vi "Get Step Information From Sequencer Configuration.vi"(10 "LstBox Refnum":refnum<vi>, 11 "Sequencer Module configuration in":refnum<class "Sequencer Module configuration.lvclass">) -> (0 "error out":errorcluster, 3 "Array":string[][](array[string]))   [LabVIEW 2015]
uses:
  module/configuration/Sequencer Module configuration.lvclass
  module/configuration/Sequencer Module configuration.lvclass/Sequencer Module configuration.ctl
  module/configuration/Read Lines.vi
  classes/Sequence/Config/Sequence Config.lvclass
  classes/Step/Config/Step Config.lvclass
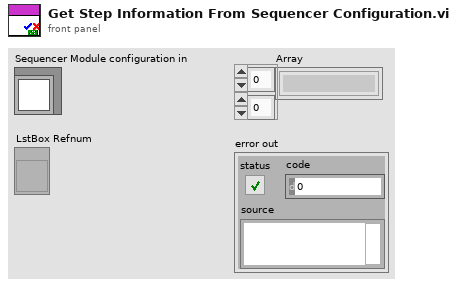
[diagram p1: front panel]
types:
  T1 = typedef "Sequencer Module configuration.lvclass/Line.ctl" = cluster{"Sequence":refnum<class "Sequence Config.lvclass">}
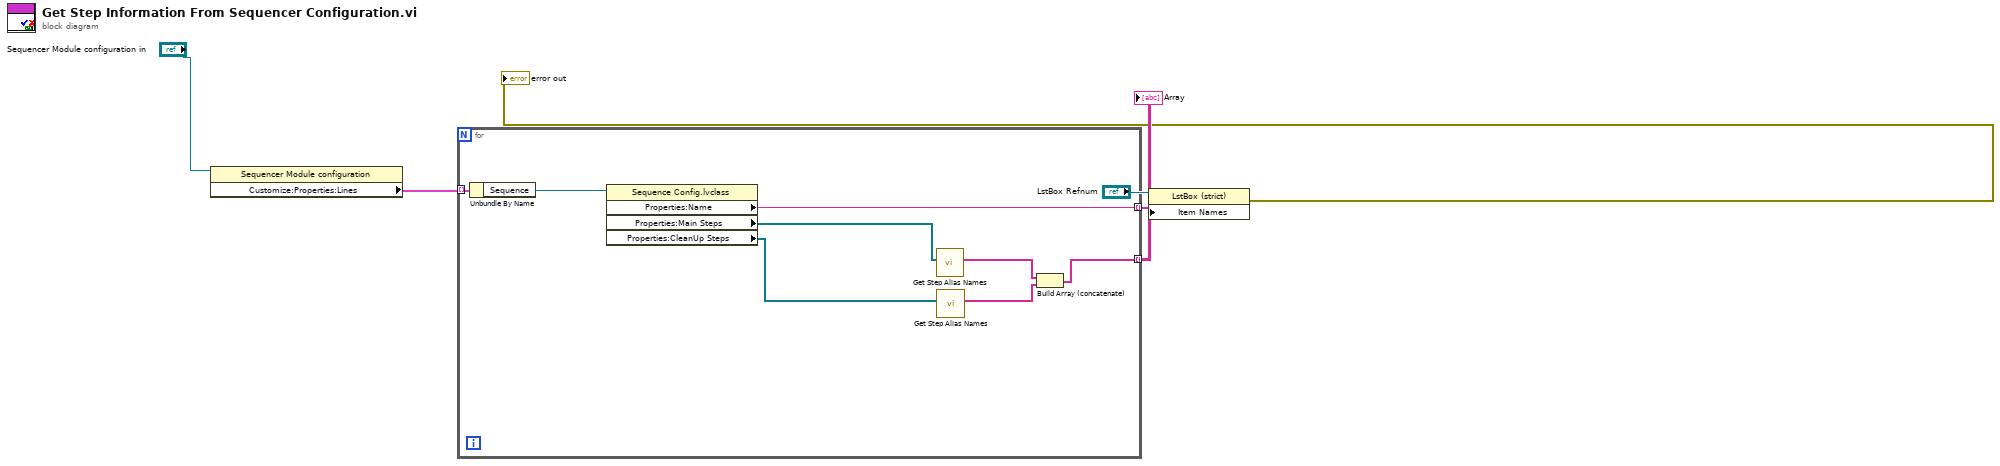
[diagram p0: block diagram]
diagram:
  n1 = property class="Sequencer Module configuration"(reference="Sequencer Module configuration in") -> ("Customize:Properties:Lines"=w3:T1[])  [unwired: 1 in, 2 out]
  n2 = for {
    tunnel: w3 -> [w14] mode=indexing
    tunnel: [w10] -> w4 mode=indexing
    tunnel: [w7] -> w6 mode=indexing
    n3 = Unbundle By Name(w14) -> ("Sequence"=w13:refnum<class "Sequence Config.lvclass">)
    n4 = property class="Sequence Config.lvclass"(reference=w13) -> ("Properties:Name"=w10:string, "Properties:Main Steps"=w12:refnum<class "Step Config.lvclass">[], "Properties:CleanUp Steps "=w11:refnum<class "Step Config.lvclass">[])  [unwired: 1 in, 2 out]
    n5 = call "Get Step Alias Names.vi"("Properties:Main Steps"=w12) -> ("Steps Alias"=w9:string[])  [unwired: 10 in]
    n6 = call "Get Step Alias Names.vi"("Properties:Main Steps"=w11) -> ("Steps Alias"=w8:string[])  [unwired: 10 in]
    n7 = Build Array (concatenate)(w9, w8) -> (w7:string[])
  }
  "Array" <- w6
  n8 = property on="Property Node" class="LstBox (strict)"(reference="LstBox Refnum", "Item Names"=w4) -> (error out=→"error out":errorcluster)  [unwired: 1 in, 1 out]
